vi "LEDC SWIR 1931 Main.vi"(0 "LEDAD Port":refnum<visa-resource-name>="COM7", 2 "Unit":u16(ring) items=["nW/cm^2", "pW/cm^2"], 5 "Light Meter Port":refnum<visa-resource-name>="COM4", 7 "Intensity Desired":dbl(slide) scale=0.0..100.0, 9 "Enable LED":u8(slide) scale=0.0..31.0, 11 "error in (no error)":errorcluster) -> (3 "In Progress":bool, 4 "LEDAD Port out":refnum<visa-resource-name>, 6 "Light Meter Port out":refnum<visa-resource-name>, 8 "Meas Illum":dbl format="%#_4g", 14 "Done":bool, 15 "error out":errorcluster)   [LabVIEW 2010]
panel:
  # "%"
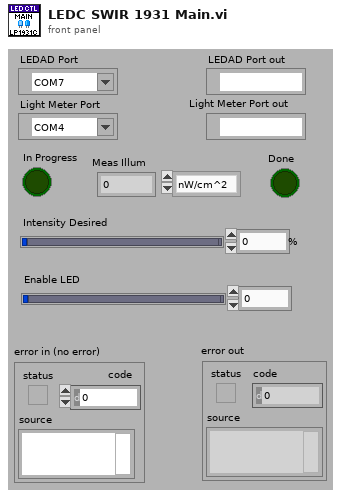
[diagram p1: front panel]
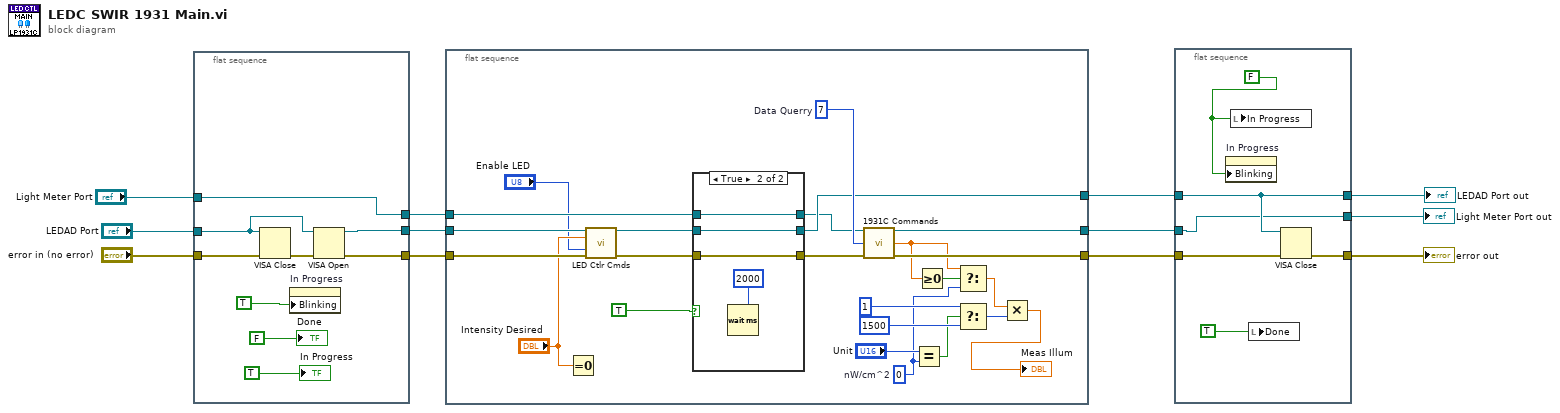
[diagram p0: block diagram]
diagram:
  n1 = flat-sequence {
    tunnel: "LEDAD Port" -> [w14]
    tunnel: [w16] -> w4
    tunnel: "error in (no error)" -> [w17]
    tunnel: [w15] -> w6
    tunnel: "Light Meter Port" -> [w13]
    tunnel: [w13] -> w5
    frame #0 {
      n2 = VISA Close(VISA resource name=w14, error in (no error)=w17) -> (error out=w18:errorcluster)
      n3 = property on="In Progress" class="Bool (strict)"("Blinking"=TRUE) -> ()  [unwired: 2 in, 2 out]
      n4 = VISA Open(error in (no error)=w18, VISA resource name=w14) -> (VISA resource name=w15:refnum<visa-resource-name>, error out=w16:errorcluster)  [unwired: 3 in]
      "Done" <- FALSE
      "In Progress" <- TRUE
    }
  }
  n5 = flat-sequence {
    tunnel: w4 -> [w26]
    tunnel: w6 -> [w28]
    tunnel: w5 -> [w31]
    tunnel: [w40] -> w12
    tunnel: [w30] -> w10
    tunnel: [w39] -> w11
    frame #0 {
      w34 = 0  # nW/cm^2
      w41 = 7  # Data Querry
      n6 = Equal To 0?(x="Intensity Desired") -> ()  [unwired: 1 out]
      n7 = call "LED Ctlr Cmds.vi"("VISA session"=w28, "Intensity"="Intensity Desired", "Enable"="Enable LED", "error in (no error)"=w26) -> ("VISA session out"=w27:refnum<visa-resource-name>, "error out"=w25:errorcluster)  [unwired: 7 in, 3 out]
      n8 = case shown="True" TRUE {
        tunnel: w25 -> [w48 w51]
        tunnel: [w48 w51] -> w32
        tunnel: [w47 w50] -> w30
        tunnel: w27 -> [w47 w50]
        tunnel: [w46 w49] -> w29
        tunnel: w31 -> [w46 w49]
        frame False {
        }
        frame True {
          n9 = Wait (ms)(milliseconds to wait=2000) -> ()  [unwired: 1 out]
        }
      }
      n10 = call "1931C Commands.vi"("Instrument Resource Name"=w29, "Command"=w41, "error in (no error)"=w32) -> ("VISA resource name out"=w40:refnum<visa-resource-name>, "LM Response"=w35:dbl, "error out"=w39:errorcluster)  [unwired: 8 in, 2 out]
      n11 = Equal?(x="Unit", y=w34) -> (x = y?=w43:bool)
      n12 = Greater Or Equal To 0?(x=w35) -> (x >= 0?=w36:bool)
      n13 = Select(t=w35, s=w36, f=w34) -> (s? t:f=w33:dbl)
      n14 = Select(t=1, s=w43, f=1500) -> (s? t:f=w42:i32)
      n15 = Multiply(x=w33, y=w42) -> (x*y=→"Meas Illum":dbl)
    }
  }
  n16 = flat-sequence {
    tunnel: w12 -> [w55]
    tunnel: w11 -> [w53]
    tunnel: [w56] -> w7
    tunnel: w10 -> [w56]
    tunnel: [w55] -> w8
    tunnel: [w54] -> w9
    frame #0 {
      w58 = FALSE
      n17 = property on="In Progress" class="Bool (strict)"("Blinking"=w58) -> ()  [unwired: 2 in, 2 out]
      n18 = local write "In Progress"(w58) -> ()
      n19 = local write "Done"(TRUE) -> ()
      n20 = VISA Close(VISA resource name=w56, error in (no error)=w53) -> (error out=w54:errorcluster)
    }
  }
  "LEDAD Port out" <- w7
  "Light Meter Port out" <- w8
  "error out" <- w9
